vi "ProdaNG.TestStep.New.vi"(8 "error in (no error)":errorcluster, 10 "TestStep":T1, 11 "dbHandleIn":i32) -> (0 "error out":errorcluster, 2 "TestStep out":T1, 3 "dbHandle":i32)   [LabVIEW 2016]
doc: "This function returns a product structure for a product, which is identified by a part and a serial number.\nImportant information: The field 'individual' was taken over from the field 'allgemein' of the legacy data directly. Because of this most products have the value 0 further on and only a few the value 1. \nParameter:\nhandle is an Integer, which is returned by the function Login() at the creation of a new connection.\nwabcoPartId is the Id of the part.\nserialNumber is the serial number of the product for the part above.\nproduct is a pointer on a product structure, which is filled if the returncode is 0. The structure must be defined in the calling program.\n\nReturncodes:\n0 No error\n< 0 ORACLE Error code\n6 (ERROR_INVALID_HANDLE) in case of an invalid handle\n1403 Record does not exist"
uses:
  Controls/ProdaNG.TestStep.ctl
  Controls/ProdaNG.TestStepSize.ctl
  Controls/ProdaNG.ReleaseId.ctl
  prodllNG.dll
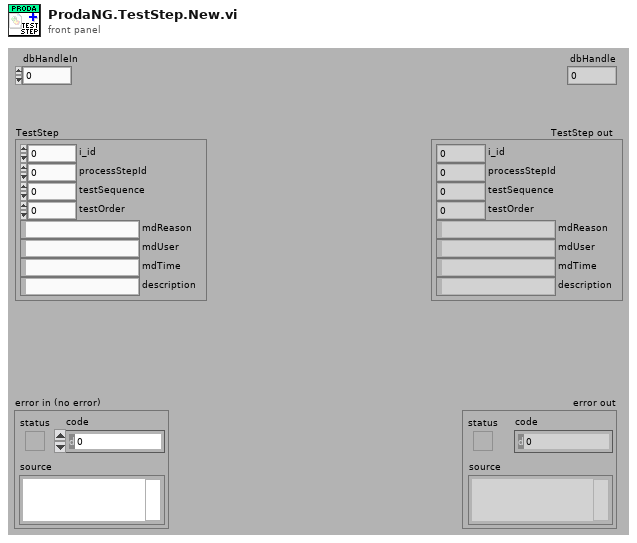
[diagram p1: front panel]
types:
  T1 = typedef "ProdaNG.TestStep.ctl" = cluster{"i_id":i32, "processStepId":i32, "testSequence":i32, "testOrder":i32, "mdReason":string, "mdUser":string, "mdTime":string, "description":string}
  T2 = typedef "ProdaNG.ReleaseId.ctl" = enum16{"not released", "released", "was released"}
  T3 = typedef "ProdaNG.TestStepSize.ctl" = cluster{"i_id":i32, "processStepId":i32, "testSequence":i32, "testOrder":i32, "mdReason":i32, "mdUser":i32, "mdTime":i32, "description":i32}
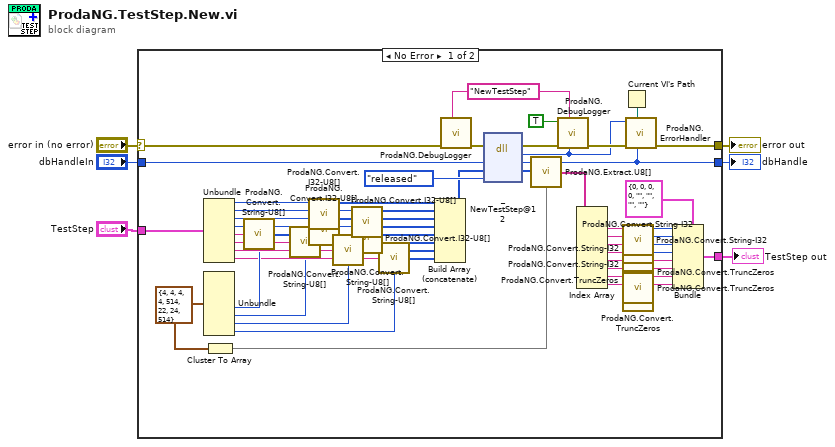
[diagram p0: block diagram]
diagram:
  n1 = case shown="No Error" "error in (no error)" {
    selector: "error in (no error)" -> [w57 w64]
    tunnel: [w62 w64] -> w5
    tunnel: "dbHandleIn" -> [w59 w63]
    tunnel: [w60 w63] -> w3
    tunnel: "TestStep" -> [w22 _]
    tunnel: [w7 _] -> w1
    frame No Error {
      w23 = T3 {"i_id"=4, "processStepId"=4, "testSequence"=4, "testOrder"=4, "mdReason"=514, "mdUser"=22, "mdTime"=24, "description"=514} ("TestStepSize")
      w53 = "NewTestStep" ("cmd")
      n2 = Unbundle(w22) -> ("i_id"=w48:i32, "processStepId"=w49:i32, "testSequence"=w18:i32, "testOrder"=w17:i32, "mdReason"=w46:string, "mdUser"=w14:string, "mdTime"=w44:string, "description"=w13:string)
      n3 = Unbundle(w23) -> ("mdReason"=w42:i32, "mdUser"=w10:i32, "mdTime"=w41:i32, "description"=w11:i32)  [unwired: 4 out]
      n4 = Cluster To Array(cluster=w23) -> (array=w19:i32[])
      n5 = call "ProdaNG.Convert.String-U8[].vi"("Input String"=w46, "Size"=w42) -> ("Output"=w45:u8[])
      n6 = call "ProdaNG.Convert.String-U8[].vi"("Input String"=w14, "Size"=w10) -> ("Output"=w8:u8[])
      n7 = call "ProdaNG.Convert.I32-U8[].vi"("32bit integer"=w48) -> ("unsigned byte array"=w47:u8[])  [unwired: 10 in]
      n8 = call "ProdaNG.Convert.I32-U8[].vi"("32bit integer"=w18) -> ("unsigned byte array"=w15:u8[])  [unwired: 10 in]
      n9 = call "ProdaNG.Convert.String-U8[].vi"("Input String"=w44, "Size"=w41) -> ("Output"=w43:u8[])
      n10 = call "ProdaNG.Convert.I32-U8[].vi"("32bit integer"=w49) -> ("unsigned byte array"=w50:u8[])  [unwired: 10 in]
      n11 = call "ProdaNG.Convert.I32-U8[].vi"("32bit integer"=w17) -> ("unsigned byte array"=w16:u8[])  [unwired: 10 in]
      n12 = call "ProdaNG.Convert.String-U8[].vi"("Input String"=w13, "Size"=w11) -> ("Output"=w12:u8[])
      n13 = Build Array (concatenate)(w47, w50, w15, w16, w45, w8, w43, w12) -> (w21:u8[])
      n14 = call "ProdaNG.DebugLogger.vi"("cmd"=w53, "error in (no error)"=w57) -> ("error out"=w56:errorcluster)  [unwired: 9 in]
      n15 = dll-call lib="D:/svn/LineTraceSystem/SOFTWARE/sources/Database/ProdaNG/prodllNG.dll" fn="_NewTestStep@12" ("ProDLL wrapper.dll:ProDLL_wrapper_GetWabcoParts_GetData")(error in=w56, "dbHandle"=w59, "testStep"=w21, "releaseId"=ProdaNG.ReleaseId."released" ("orderby (Test Sequence)")) -> (error out=w55:errorcluster, "return type"=w52:i32, "dbHandle"=w60:i32, "testStep"=w20:u8[])  [unwired: 3 in, 1 out]
      n16 = call "ProdaNG.Extract.U8[].vi"("unsigned byte array"=w20, "Sizes"=w19) -> ("Elements"=w40:string[])
      n17 = call "ProdaNG.DebugLogger.vi"("return type"=w52, "cmd"=w53, "error in (no error)"=w55, "done? (F)"=TRUE) -> ("error out"=w54:errorcluster)  [unwired: 7 in]
      n18 = Index Array(array=w40) -> (element #1=w39:string, element #2=w36:string, element #3=w35:string, element #4=w29:string, element #5=w26:string, element #6=w25:string, element #7=w30:string, element #8=w32:string)  [unwired: 8 in]
      n19 = Current VI's Path() -> (path=w61:path)
      n20 = call "ProdaNG.Convert.String-I32.vi"("unsigned byte string"=w39) -> ("32bit integer"=w38:i32)  [unwired: 10 in]
      n21 = call "ProdaNG.Convert.String-I32.vi"("unsigned byte string"=w36) -> ("32bit integer"=w37:i32)  [unwired: 10 in]
      n22 = call "ProdaNG.Convert.String-I32.vi"("unsigned byte string"=w35) -> ("32bit integer"=w34:i32)  [unwired: 10 in]
      n23 = call "ProdaNG.Convert.String-I32.vi"("unsigned byte string"=w29) -> ("32bit integer"=w28:i32)  [unwired: 10 in]
      n24 = call "ProdaNG.Convert.TruncZeros.vi"("string with \\0s"=w26) -> ("LV string"=w27:string)  [unwired: 10 in]
      n25 = call "ProdaNG.Convert.TruncZeros.vi"("string with \\0s"=w25) -> ("LV string"=w24:string)  [unwired: 10 in]
      n26 = call "ProdaNG.Convert.TruncZeros.vi"("string with \\0s"=w30) -> ("LV string"=w31:string)  [unwired: 10 in]
      n27 = call "ProdaNG.Convert.TruncZeros.vi"("string with \\0s"=w32) -> ("LV string"=w33:string)  [unwired: 10 in]
      n28 = call "ProdaNG.ErrorHandler.vi"("dbHandleIn"=w60, "Path"=w61, "error in"=w54, "output_parameter"=w52) -> ("error out"=w62:errorcluster)  [unwired: 7 in]
      n29 = Bundle(cluster=T1 {"i_id"=0, "processStepId"=0, "testSequence"=0, "testOrder"=0, "mdReason"="", "mdUser"="", "mdTime"="", "description"=""} ("TestStep"), "i_id"=w38, "processStepId"=w37, "testSequence"=w34, "testOrder"=w28, "mdReason"=w27, "mdUser"=w24, "mdTime"=w31, "description"=w33) -> (w7:T1)
    }
    frame Error {
    }
  }
  "error out" <- w5
  "dbHandle" <- w3
  "TestStep out" <- w1
